vi "Actor Core.vi"(8 "error in":errorcluster, 11 "UDP Service in":refnum<class "UDP Service.lvclass">) -> (0 "error out":errorcluster, 3 "Actor out":refnum<class "Actor.lvclass">)   [LabVIEW 2016, in "Assert API Components.lvlib" / "UDP Service.lvlib" / "UDP Service.lvclass"]
doc: "(<B>Filename</B>: Actor Framework.lvlib:Actor.lvclass:Actor Core.vi)\n\nReceives messages to the actor, reacts to them, and initiates any error handling that may shut the actor down.\n\nDescendant classes may override this VI to append parallel tasks for the actor to complete while it handles messages. Overrides use the Call Parent Method node."
uses:
  UDP Service.lvclass
  D:/Work/Projects/actor_assert_api/Core/Base UI Actor/Base UI Actor/Base UI Actor.lvclass
  C:/Program Files (x86)/National Instruments/LabVIEW 2016/vi.lib/ActorFramework/Actor/Actor.lvclass
  <vilib>/ActorFramework/Actor/Actor.lvclass
  <vilib>/ActorFramework/Actor/Actor.lvclass/Actor.ctl
  Base UI Actor/Base UI Actor/Base UI Actor.lvclass/Base UI Actor.ctl
  UDP Service.lvclass/UDP Service.ctl
  Main Display/Main Display Messages/New Assert Message Msg/New Assert Message Msg.lvclass/New Assert Message Msg.ctl
  <vilib>/ActorFramework/Message Enqueuer/Message Enqueuer.lvclass/Message Enqueuer.ctl
  <vilib>/ActorFramework/Message Enqueuer/Enqueue.vi
  Main Display/Main Display Messages/New Assert Message Msg/New Assert Message Msg.lvclass
  C:/Program Files (x86)/National Instruments/LabVIEW 2016/vi.lib/ActorFramework/Message/Message.lvclass
  <vilib>/ActorFramework/Message Priority Queue/Priority Enqueue.vi
  Base UI Actor/Base UI Actor/Base UI Actor.lvclass
panel:
  out "IP Address":string
  out "Service Name":string
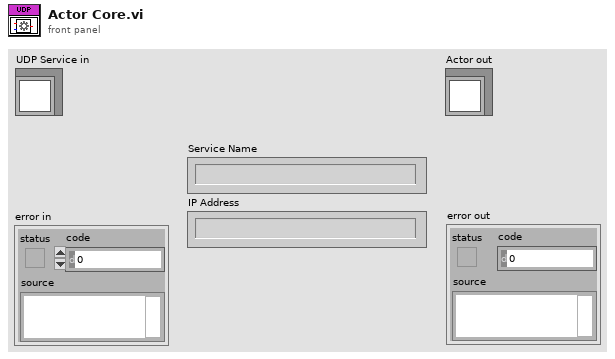
[diagram p1: front panel]
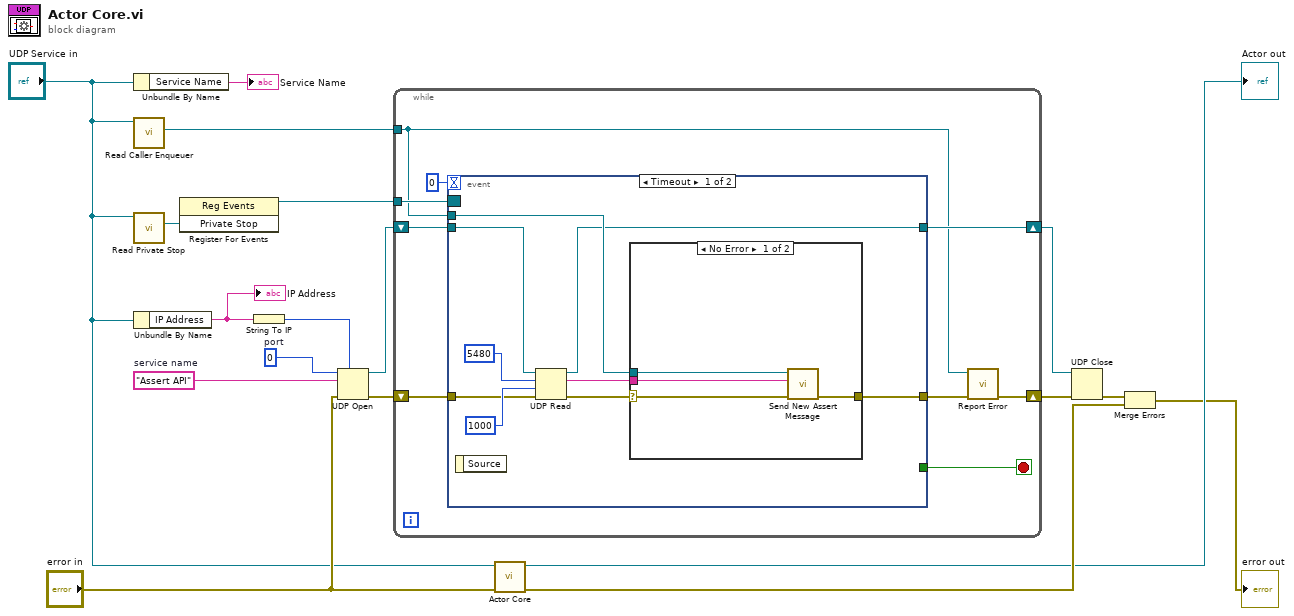
[diagram p0: block diagram]
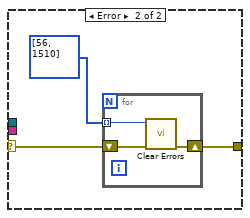
[diagram p2: hidden frame]
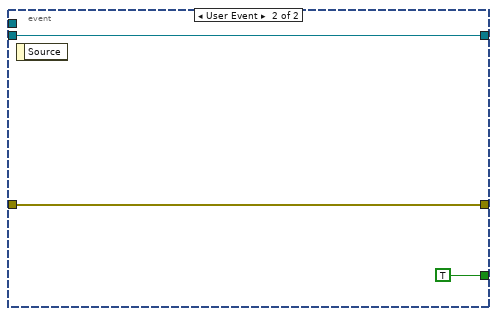
[diagram p3: hidden frame]
diagram:
  w4 = "Assert API"  # service name
  w13 = u16 0  # port
  n1 = Unbundle By Name("UDP Service in") -> ("Service Name"=→"Service Name":string)
  n2 = call <vilib>:"Read Caller Enqueuer.vi"("Actor"="UDP Service in") -> ("Caller Enqueuer"=w9:refnum<class "Message Enqueuer.lvclass">)  [unwired: 10 in]
  n3 = call "Read Private Stop.vi"("Base UI Actor in"="UDP Service in") -> ("Private Stop"=w16:refnum<user-event>)  [unwired: 10 in]
  n4 = Unbundle By Name("UDP Service in") -> ("IP Address"=w2:string)
  "IP Address" <- w2
  n5 = register-events(w16) -> (reference out=w15:refnum<event-registration>)  [unwired: 2 in, 1 out]
  n6 = String To IP(1:w2) -> (0:w3:u32)
  n7 = UDP Open(7:w3, 8:"error in", 10:w4, 11:w13) -> (port=w11:refnum<k16>, 0:w10:errorcluster)  [unwired: 1 in, 1 out]
  n8 = while {
    tunnel: w15 -> [w27]
    tunnel: w9 -> [w21]
    shift-right: [w22] -> w6
    shift-left: w11 -> [w24]
    shift-right: [w19] -> w8
    shift-left: w10 -> [w23]
    stop <- w25 stop-if-true
    n9 = event shown="[0] Timeout" {
      selector: w27 -> [_ _]
      dyn-events: _ -> [_ _]
      timeout: 0 -> [_ _]
      tunnel: [_ TRUE] -> w25
      tunnel: w24 -> [w32 w47]
      tunnel: w23 -> [w31 w48]
      tunnel: w21 -> [w30 _]
      tunnel: [w29 w48] -> w20
      tunnel: [w28 w47] -> w22
      event Timeout {
        n10 = event-data() -> ()  [unwired: 1 in, 1 out]
        n11 = UDP Read(connection ID=w32, max size (548)=5480, timeout ms (25000)=1000, 8:w31) -> (data out=w34:string, error out=w33:errorcluster, 3:w28:refnum<k16>)  [unwired: 2 out]
        n12 = case shown="No Error" w33 {
          selector: w33 -> [w39 w42]
          tunnel: [w40 w41] -> w29
          tunnel: w34 -> [w38 _]
          tunnel: w30 -> [w37 _]
          frame No Error {
            n13 = call "Send New Assert Message.vi"("error in (no error)"=w39, "Assert Message"=w38, "Message Enqueuer"=w37) -> ("error out"=w40:errorcluster)  [unwired: 7 in, 1 out]
          }
          frame Error {
            n14 = for {
              tunnel: i32[] [56, 1510] ("specific error code to clear (0: all)") -> [w46] mode=indexing
              shift-right: [w44] -> w41
              shift-left: w42 -> [w45]
              n15 = call <vilib>:"Clear Errors.vi"("error in (no error)"=w45, "specific error code to clear (0: all)"=w46) -> ("error out"=w44:errorcluster)  [unwired: 4 in, 1 out]
            }
          }
        }
      }
      event User Event {
        n16 = event-data() -> ()  [unwired: 1 in, 1 out]
      }
    }
    n17 = call "Report Error.vi"("error in (no error)"=w20, "Self Enqueuer"=w21) -> ("error out"=w19:errorcluster)  [unwired: 9 in]
  }
  n18 = call-parent "Actor Core.vi"("error in"="error in", "Actor in"="UDP Service in") -> ("error out"=w18:errorcluster, "Actor out"=→"Actor out":refnum<class "Actor.lvclass">)  [unwired: 8 in]
  n19 = UDP Close(connection ID=w6, 8:w8) -> (error out=w7:errorcluster)  [unwired: 1 out]
  n20 = Merge Errors(w7, w18) -> (→"error out":errorcluster)
